vi "Startup Main.vi"(6 "LabVIEW Web Service":refnum<class "Web Service.lvclass">) -> ()   [LabVIEW 2020]
uses:
  <vilib>/wsapi/Web Service.lvclass
  <userlib>/_NEVSTOP/Communicable State Machine(CSM)/addons/Watchdog/CSM Watchdog.lvlib
panel:
  # "Use the web service input terminal to call the VIs on the Service subpalette of the Web Services palette. Do not remove it from the connector pane unless you don't need access to the palette."
  # "Any additional terminals added to the connector pane of a startup VI will be ignored."
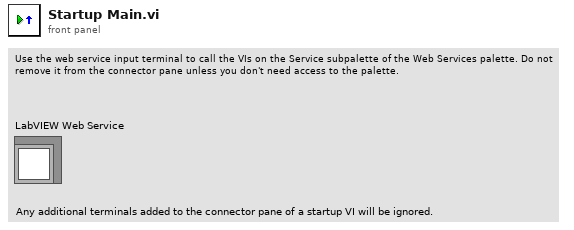
[diagram p1: front panel]
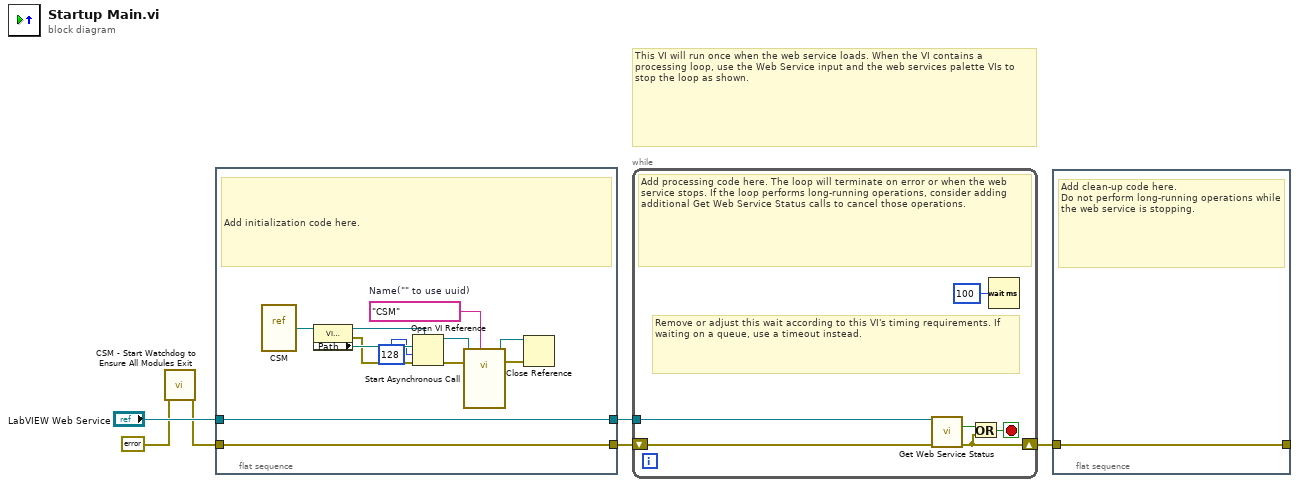
[diagram p0: block diagram]
diagram:
  # "This VI will run once when the web service loads. When the VI contains a processing loop, use the Web Service input and the web services palette VIs to stop the loop as shown."
  n1 = call <userlib>:"CSM - Start Watchdog to Ensure All Modules Exit.vi"("error in (no error)"=errorcluster {"status"=FALSE, "code"=0, "source"=""} ("error constant")) -> ("error out"=w1:errorcluster)  [unwired: 10 in]
  n2 = flat-sequence {
    tunnel: "LabVIEW Web Service" -> [w18]
    tunnel: [w18] -> w5
    tunnel: [w17] -> w4
    tunnel: w1 -> [w17]
    frame #0 {
      w7 = "CSM"  # Name("" to use uuid)
      # "Add initialization code here."
      n3 = vi-ref "CSM.vi"() -> (w15:refnum<vi>)
      n4 = property class="VI (strict)"(reference=w15) -> (reference out=w11:refnum<vi>, error out=w13:errorcluster, "Path"=w14:path)  [unwired: 1 in]
      n5 = Open VI Reference(type specifier VI Refnum (for type only)=w11, vi path=w14, options=128, error in (no error)=w13) -> (vi reference=w12:refnum<vi>, error out=w16:errorcluster)  [unwired: 2 in]
      n6 = call-by-ref "Start Asynchronous Call"(reference=w12, error in=w16, "Name(\"\" to use uuid)"=w7) -> (reference out=w9:refnum<vi>, error out=w10:errorcluster)  [unwired: 11 in]
      n7 = Close Reference(reference=w9, error in (no error)=w10) -> ()  [unwired: 1 out]
    }
  }
  n8 = while {
    tunnel: w5 -> [w23]
    shift-right: [w20] -> w2
    shift-left: w4 -> [w21]
    stop <- w22 stop-if-true
    # "Remove or adjust this wait according to this VI's timing requirements. If waiting on a queue, use a timeout instead."
    # "Add processing code here. The loop will terminate on error or when the web service stops. If the loop performs long-running operations, consider adding additional Get Web Service Status calls to cancel those operations."
    n9 = call <vilib>:"Get Web Service Status.vi"("LabVIEW Web Service"=w23, "error in (no error)"=w21) -> ("service stopping?"=w24:bool, "error out"=w20:errorcluster)  [unwired: 11 in, 1 out]
    n10 = Or(x=w24, y=w20) -> (x .or. y?=w22:bool)
    n11 = Wait (ms)(milliseconds to wait=u32 100) -> ()  [unwired: 1 out]
  }
  n12 = flat-sequence {
    tunnel: [w25] -> _
    tunnel: w2 -> [w25]
    frame #0 {
      # "Add clean-up code here.\nDo not perform long-running operations while the web service is stopping."
    }
  }
